vi "ziCpuProgram.vi"(3 "error in":errorcluster, 4 "device (active)":string, 5 "Filename":string, 6 "Handle In":T1 {"Handle" format="0x%08x"; "Conn" format="0x%08x"}) -> (0 "error out":errorcluster, 2 "Handle Out":T1 {"Handle" format="0x%08x"; "Conn" format="0x%08x"})   [LabVIEW 2009, in "Zurich Instruments LabOne.lvlib"]
doc: "This vi programs the RT option of an HF2 Series instrument"
uses:
  <instrlib>/Zurich Instruments LabOne/Zurich Instruments LabOne.lvlib
  <instrlib>/Zurich Instruments LabOne/Public/ziTypeHandle.ctl
  <instrlib>/Zurich Instruments LabOne/Private/ziLV32.dll
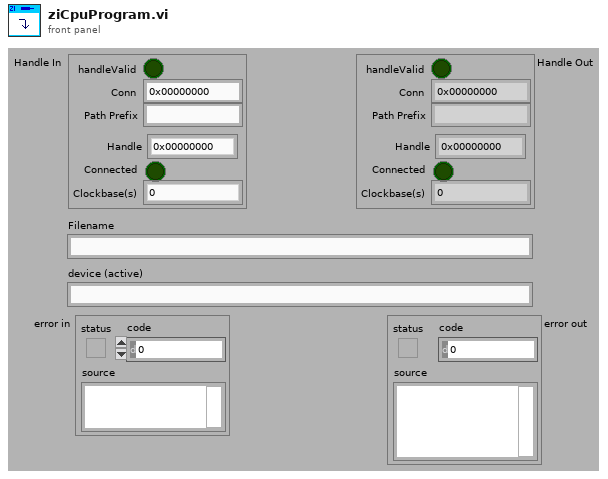
[diagram p1: front panel]
types:
  T1 = typedef "Zurich Instruments LabOne.lvlib/ziTypeHandle.ctl" = cluster{"handleValid":bool, "Conn":u64, "Path Prefix":string, "Handle":u64, "Connected":bool, "Clockbase(s)":dbl}
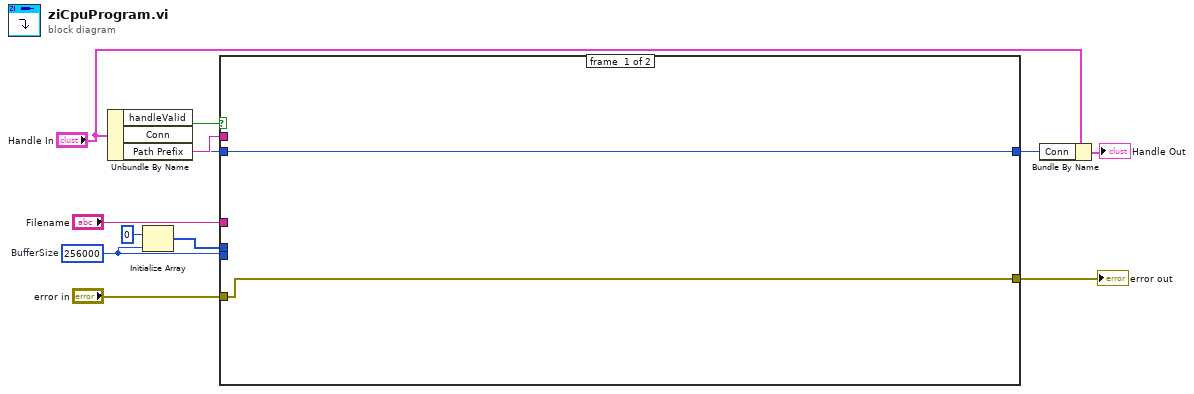
[diagram p0: block diagram]
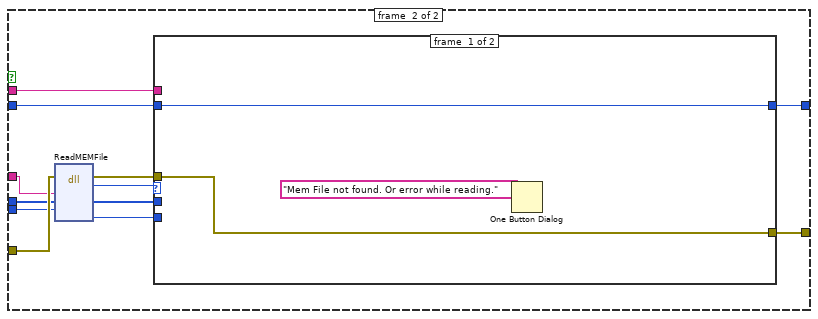
[diagram p2: hidden frame]
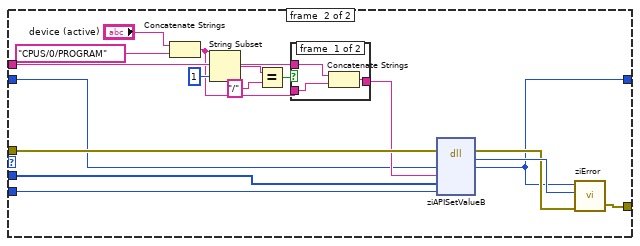
[diagram p3: hidden frame]
diagram:
  w5 = 256000  # BufferSize
  n1 = Unbundle By Name("Handle In") -> ("handleValid"=w6:bool, "Conn"=w8:u64, "Path Prefix"=w10:string)
  n2 = Initialize Array(u8 0 ("element"), w5) -> (w3:u8[])
  n3 = case shown="True" w6 {
    tunnel: "error in" -> [w13 w26]
    tunnel: w5 -> [_ w25]
    tunnel: [w13 w24] -> w11
    tunnel: w10 -> [_ w23]
    tunnel: "Filename" -> [_ w22]
    tunnel: w8 -> [w14 w20]
    tunnel: [w14 w17] -> w7
    tunnel: w3 -> [_ w15]
    frame #0 {
    }
    frame #1 {
      n4 = dll-call lib="C:/Program Files (x86)/National Instruments/LabVIEW 2009/instr.lib/Zurich Instruments LabOne/Private/ziLV*.*" fn="ReadMEMFile"(error in=w26, "Filename"=w22, "Buffer"=w15, "BuffeSize"=w25) -> (error out=w21:errorcluster, "return type"=w16:u32, "Buffer"=w19:u8[], "bytesUsed"=w18:u32)  [unwired: 4 in, 2 out]
      n5 = case shown="0" w16 {
        tunnel: [w27 w46] -> w24
        tunnel: w23 -> [_ w41]
        tunnel: w21 -> [w27 w40]
        tunnel: w20 -> [w29 w38]
        tunnel: w19 -> [_ w37]
        tunnel: w18 -> [_ w36]
        tunnel: [w29 w30] -> w17
        frame #0 {
          n6 = One Button Dialog(message="Mem File not found. Or error while reading.") -> ()  [unwired: 2 out]
        }
        frame #1 {
          n7 = Concatenate Strings("device (active)", "CPUS/0/PROGRAM") -> (w31:string)
          n8 = String Subset(string=w31, length (rest)=1 ("length (rest)")) -> (substring=w44:string)  [unwired: 1 out]
          n9 = Equal?(x=w44, y="/") -> (x = y?=w42:bool)
          n10 = case shown="False" w42 {
            tunnel: w41 -> [w47 _]
            tunnel: [w49 w50] -> w39
            tunnel: w31 -> [w48 w50]
            frame #0 {
              n11 = Concatenate Strings(w47, w48) -> (w49:string)
            }
            frame #1 {
            }
          }
          n12 = dll-call lib="C:/Program Files (x86)/National Instruments/LabVIEW 2009/instr.lib/Zurich Instruments LabOne/Private/ziLV*.*" fn="ziAPISetValueB"(error in=w40, "Conn"=w38, "Path"=w39, "Buffer"=w37, "Len"=w36) -> (error out=w34:errorcluster, "return type"=w35:u32, "Conn"=w30:u64)  [unwired: 5 in, 1 out]
          n13 = call <instrlib>:"ziError.vi"("Conn"=w30, "ziErrorCode"=w35, "Error In"=w34) -> ("Error Out"=w46:errorcluster)  [unwired: 2 in, 1 out]
        }
      }
    }
  }
  "error out" <- w11
  n14 = Bundle By Name(cluster="Handle In", "Conn"=w7) -> (→"Handle Out":T1)
